vi "isSelectedDisabled.vi"(8 "error in (no error)":errorcluster, 11 "GoalListUIAdapter in":refnum<class "SingleSelectMCLBAdapter.lvclass">) -> (0 "error out":errorcluster, 2 "Disabled?":bool, 3 "GoalListUIAdapter out":refnum<class "SingleSelectMCLBAdapter.lvclass">)   [LabVIEW 2020, in "SingleSelectMCLBAdapter.lvclass"]
uses:
  SingleSelectMCLBAdapter.lvclass
  <vilib>/Utility/miscctls.llb/LVRowAndColumnTypeDef.ctl
  SingleSelectMCLBAdapter.lvclass/SingleSelectMCLBAdapter.ctl
  AbstractMultiColumnListBoxAdapter/AbstractMultiColumnListBoxAdapter.lvclass
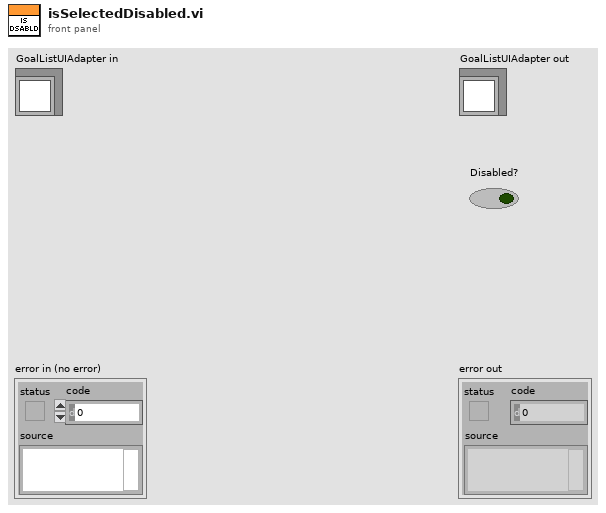
[diagram p1: front panel]
types:
  T1 = typedef "LVRowAndColumnTypeDef.ctl" = cluster{"Row":i32, "Column":i32}
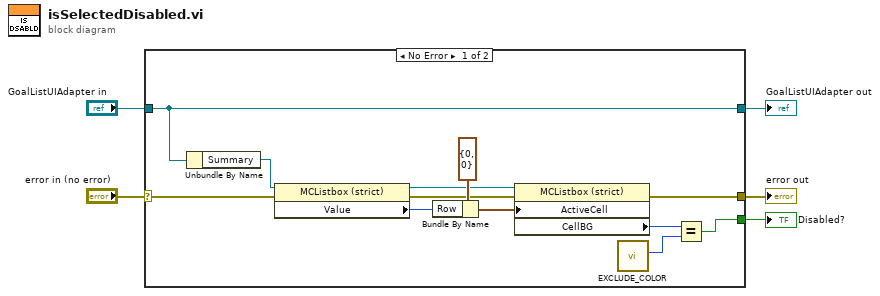
[diagram p0: block diagram]
diagram:
  n1 = case shown="No Error" "error in (no error)" {
    selector: "error in (no error)" -> [w10 w19]
    tunnel: [w9 w19] -> w4
    tunnel: [w8 w18] -> w2
    tunnel: "GoalListUIAdapter in" -> [w8 w18]
    tunnel: [w13 _] -> w1
    frame No Error {
      n2 = Unbundle By Name(w8) -> ("Summary"=w7:refnum<vi>)
      n3 = property class="MCListbox (strict)"(reference=w7, error in=w10) -> (reference out=w6:refnum<vi>, error out=w12:errorcluster, "Value"=w11:i32)
      n4 = Bundle By Name(cluster=T1 {"Row"=0, "Column"=0} ("Active Cell:Active Cell"), "Row"=w11) -> (w16:T1)
      n5 = property class="MCListbox (strict)"(reference=w6, error in=w12, "ActiveCell"=w16) -> (error out=w9:errorcluster, "CellBG"=w15:u32)  [unwired: 1 out]
      n6 = call "EXCLUDE_COLOR.vi"() -> ("Color Box"=w14:u32)  [unwired: 11 in]
      n7 = Equal?(x=w15, y=w14) -> (x = y?=w13:bool)
    }
    frame Error {
    }
  }
  "error out" <- w4
  "GoalListUIAdapter out" <- w2
  "Disabled?" <- w1
